vi "Servo Tracking State Machinev1.vi"(0 "Servo Positions In":cluster{"X":dbl, "Y":dbl}, 1 "Image Size":T4=enum."320x240", 5 "Target":T1, 7 "Area Limit":dbl=0.005, 9 "Found":bool) -> (4 "Servo Positions":cluster{"X":dbl, "Y":dbl}, 6 "Tracking State Info":T3)   [LabVIEW 2013]
doc: "This VI updates the servo to center the camera on the target. It uses a state based control approach to locate follow, and reacquire the target."
uses:
  <vilib>/Rock Robotics/WPI/Camera/WPI_CameraImageSize.ctl
  Control Statesv1.ctl
panel:
  in  "Upper Limit":cluster{"X":i32, "Y":i32}={"X"=169, "Y"=130}
  in  "Lower Limit":cluster{"X":i32, "Y":i32}={"X"=0, "Y"=40}
  in  "Search Speed":i32=4
  in  "Proportional (div)":cluster{"X":i32, "Y":i32}={"X"=15, "Y"=-13}
  # "Unwired tuning params for control.\nSearch speed determines how fast the\ngimbal will move when trying to acquire\na target. Too fast and you may miss the\ntarget between frames, too slow is boring.\n\nProportional(div) is the proportional constant\nexpressed as a divisor term. Adjust this higher\nif the gimbal is oscillating, lower for quicker\nresponse.\n\nThe limits are useful for keeping the gimbal in\na working range, some stick when the get near\ntheir mechanical limits. It is also useful to limit\nthe searching to avoid looking at the ceiling, etc."
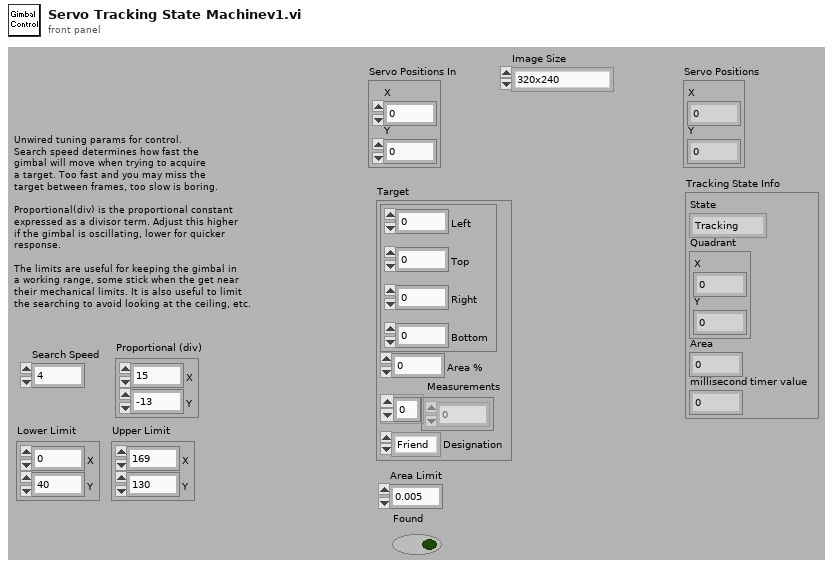
[diagram p1: front panel]
types:
  T1 = cluster{"Rectangle":cluster{"Left":i32, "Top":i32, "Right":i32, "Bottom":i32}, "Area %":dbl, "Measurements":dbl[], "Designation":enum16{"Friend", "Foe"}}
  T2 = typedef "Control Statesv1.ctl" = enum16{"Tracking", "Lost Small", "Lost-Patience", "Search-Begin", "Searching", "Lost - Edge"}
  T3 = cluster{"State":T2, "Quadrant":cluster{"X":i32, "Y":i32}, "Area":dbl, "millisecond timer value":u32}
  T4 = typedef "WPI_CameraImageSize.ctl" = enum16{"640x480", "320x240", "160x120"}
  T5 = cluster{"State":T2, "Grid Element":cluster{"X":i32, "Y":i32}, "Area":dbl, "millisecond timer value":u32}
  T6 = cluster{"Left":i32, "Top":i32, "Right":i32, "Bottom":i32}
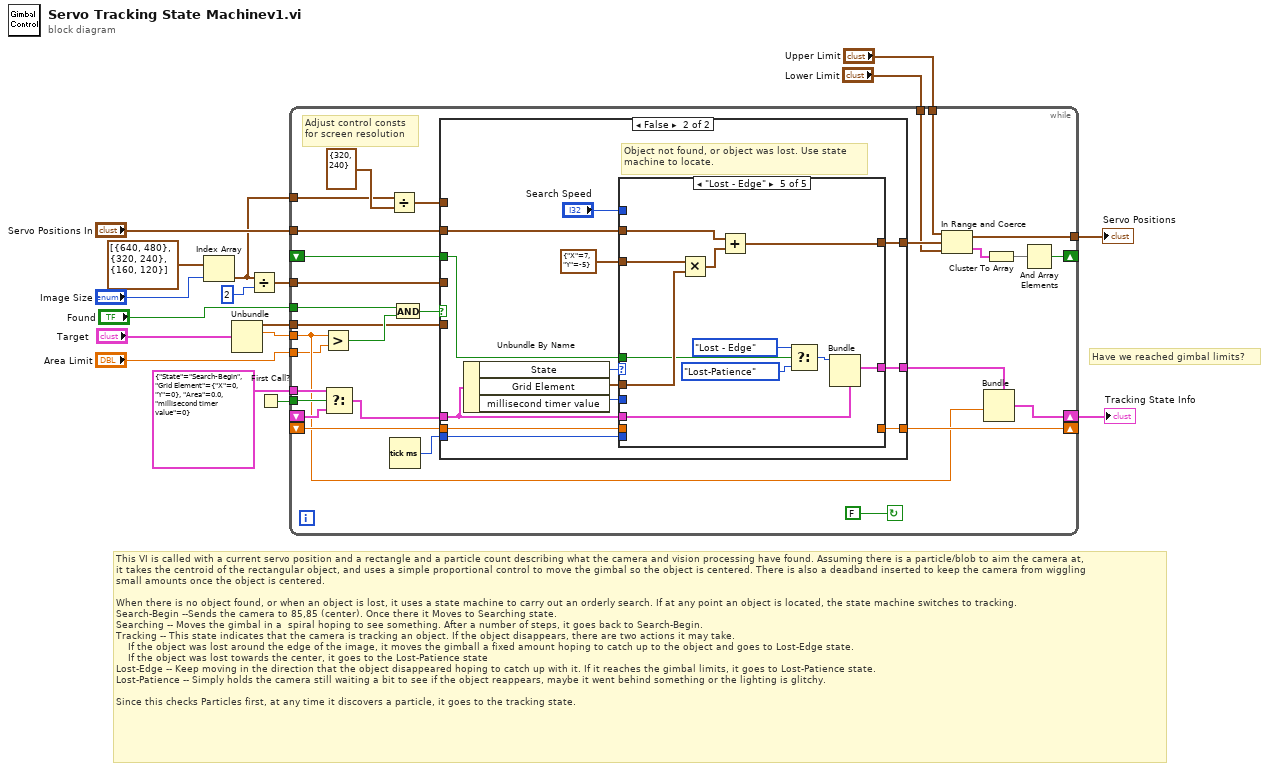
[diagram p0: block diagram]
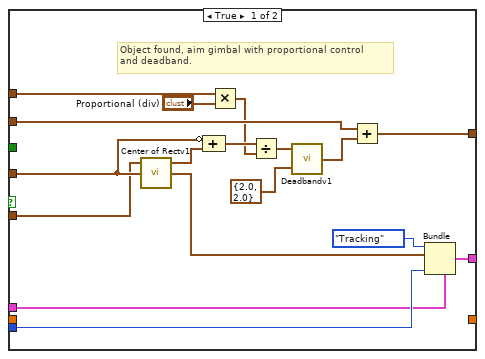
[diagram p2: hidden frame]
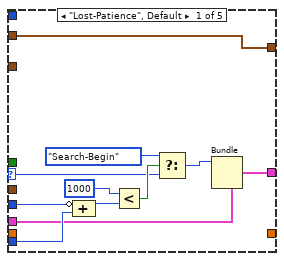
[diagram p3: hidden frame]
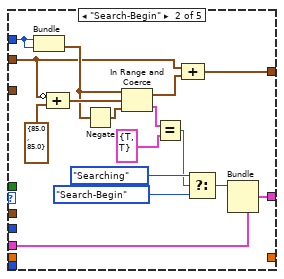
[diagram p4: hidden frame]
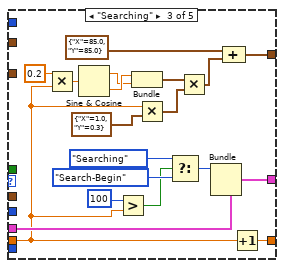
[diagram p5: hidden frame]
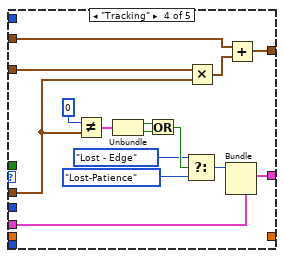
[diagram p6: hidden frame]
diagram:
  # "Have we reached gimbal limits?"
  # "This VI is called with a current servo position and a rectangle and a particle count describing what the camera and vision processing have found. Assuming there is a particle/blob to aim the camera at,\nit takes the centroid of the rectangular object, and uses a simple proportional control to move the gimbal so the object is centered. There is also a deadband inserted to keep the camera from wiggling\nsmall amounts once the object is centered.\n\nWhen there is no object found, or when an object is lost, it uses a state machine to carry out an orderly search. If at any point an object is located, the state machine switches to tracking.\nSearch-Begin --Sends the camera to 85,85 (center). Once there it Moves to Searching state.\nSearching -- Moves the gimbal in a  spiral hoping to see something. After a number of steps, it goes back to Search-Begin.\nTracking -- This state indicates that the camera is tracking an object. If the object disappears, there are two actions it may take.\n    If the object was lost around the edge of the image, it moves the gimball a fixed amount hoping to catch up to the object and goes to Lost-Edge state.\n    If the object was lost towards the center, it goes to the Lost-Patience state\nLost-Edge -- Keep moving in the direction that the object disappeared hoping to catch up with it. If it reaches the gimbal limits, it goes to Lost-Patience state.\nLost-Patience -- Simply holds the camera still waiting a bit to see if the object reappears, maybe it went behind something or the lighting is glitchy.\n\nSince this checks Particles first, at any time it discovers a particle, it goes to the tracking state."
  n1 = Index Array(array=cluster{"X":i32, "Y":i32}[] [{"X"=640, "Y"=480}, {"X"=320, "Y"=240}, {"X"=160, "Y"=120}] ("Resolutions"), index="Image Size") -> (element=w3:cluster{"X":i32, "Y":i32})
  n2 = Unbundle("Target") -> ("Rectangle"=w5:T6, "Area %"=w6:dbl)  [unwired: 2 out]
  n3 = Divide(x=w3, y=2) -> (x/y=w15:cluster{"X":dbl, "Y":dbl})
  n4 = First Call?() -> (First Call?: T/F=w10:bool)
  n5 = while {
    tunnel: w15 -> [w29]
    tunnel: [w37] -> w13
    shift-right: [w45] -> _
    shift-left: _ -> [w44]
    tunnel: "Servo Positions In" -> [w43]
    shift-right: [w26] -> w11
    shift-left: _ -> [w40]
    tunnel: w10 -> [w42]
    tunnel: T5 {"State"=enum."Search-Begin", "Grid Element"={"X"=0, "Y"=0}, "Area"=0.0, "millisecond timer value"=0} -> [w41]
    tunnel: "Lower Limit" -> [w35]
    tunnel: "Upper Limit" -> [w34]
    shift-right: [w31] -> _
    shift-left: _ -> [w30]
    tunnel: w6 -> [w24]
    tunnel: w5 -> [w23]
    tunnel: "Area Limit" -> [w22]
    tunnel: w3 -> [w19]
    tunnel: "Found" -> [w18]
    stop <- FALSE continue-if-true
    # "Adjust control consts\nfor screen resolution"
    n6 = Greater?(x=w24, y=w22) -> (0:w28:bool)
    n7 = Select(t=w41, s=w42, f=w40) -> (s? t:f=w39:T5)
    n8 = Divide(x=w19, y=cluster{"X":i32, "Y":i32} {"X"=320, "Y"=240} ("element")) -> (x/y=w21:cluster{"X":dbl, "Y":dbl})
    n9 = Tick Count (ms)() -> (millisecond timer value=w46:u32)
    n10 = And(x=w18, y=w28) -> (x .and. y?=w27:bool)
    n11 = case shown="False" w27 {
      tunnel: w29 -> [w51 _]
      tunnel: w46 -> [w59 w75]
      tunnel: [w61 w76] -> w25
      tunnel: w39 -> [w54 w68]
      tunnel: w43 -> [w60 w73]
      tunnel: [w58 w74] -> w36
      tunnel: w44 -> [_ w72]
      tunnel: [_ w71] -> w45
      tunnel: w30 -> [_ w70]
      tunnel: w23 -> [w50 _]
      tunnel: w21 -> [w47 _]
      frame True {
        # "Object found, aim gimbal with proportional control\nand deadband."
        n12 = call "Center of Rectv1.vi"("Camera Center"=w51, "Rectangle"=w50) -> ("Grid Element"=w52:cluster{"X":i32, "Y":i32}, "Center"=w53:cluster{dbl, dbl})  [unwired: 1 in, 1 out]
        n13 = Compound Arithmetic op=ADD(invert w51, w53) -> (w63:cluster{dbl, dbl})
        n14 = Multiply(x=w47, y="Proportional (div)") -> (x*y=w48:cluster{"X":dbl, "Y":dbl})
        n15 = Divide(x=w63, y=w48) -> (x/y=w56:cluster{dbl, dbl})
        n16 = call "Deadbandv1.vi"("Deadband"=cluster{dbl, dbl} {2.0, 2.0}, "Value"=w56) -> ("Value Out"=w55:cluster{dbl, dbl})
        n17 = Add(x=w60, y=w55) -> (x+y=w58:cluster{dbl, dbl})
        n18 = Bundle(cluster=w54, "State"=Control_Statesv1."Tracking", "Grid Element"=w52, "millisecond timer value"=w59) -> (w61:T5)  [unwired: 1 out]
      }
      frame False {
        # "Object not found, or object was lost. Use state\nmachine to locate."
        n19 = Unbundle By Name(w68) -> ("State"=w67:T2, "Grid Element"=w66:cluster{"X":i32, "Y":i32}, "millisecond timer value"=w65:u32)
        n20 = case shown="\"Lost - Edge\"" w67 {
          selector: w67 -> [w78 _ _ _ _]
          tunnel: [w79 w94 w109 w137 w148] -> w76
          tunnel: w68 -> [w83 w95 w110 w136 w147]
          tunnel: w65 -> [w86 _ _ _ _]
          tunnel: w75 -> [w87 _ _ _ _]
          tunnel: [w77 w96 w114 w128 w144] -> w74
          tunnel: w73 -> [w77 w97 _ w127 w145]
          tunnel: "Search Speed" -> [_ w101 _ _ _]
          tunnel: w72 -> [_ _ w105 _ _]
          tunnel: [_ _ w122 _ _] -> w71
          tunnel: w66 -> [_ _ _ w125 w143]
          tunnel: w70 -> [_ _ _ _ w139]
          tunnel: cluster{"X":i32, "Y":i32} {"X"=7, "Y"=-5} ("x") -> [_ _ _ w123 w138]
          frame "Lost-Patience", Default {
            n21 = Compound Arithmetic op=ADD(invert w86, w87) -> (w85:u32)
            n22 = Less?(x=1000, y=w85) -> (x < y?=w80:bool)
            n23 = Select(t=Control_Statesv1."Search-Begin" ("State"), s=w80, f=w78) -> (s? t:f=w82:T2)
            n24 = Bundle(cluster=w83, "State"=w82) -> (w79:T5)  [unwired: 3 out]
          }
          frame "Search-Begin" {
            n25 = Bundle("Search Speed"=w101, "Search Speed"=w101) -> (w100:cluster{"Search Speed":i32, "Search Speed":i32})  [unwired: 1 out]
            n26 = Compound Arithmetic op=ADD(invert w97, cluster{"X":dbl, "Y":dbl} {"X"=85.0, "Y"=85.0} ("Servos")) -> (w102:cluster{"X":dbl, "Y":dbl})
            n27 = Negate(x=w100) -> (-x=w99:cluster{"Search Speed":i32, "Search Speed":i32})
            n28 = In Range and Coerce(upper limit=w100, x=w102, lower limit=w99) -> (coerced(x)=w98:cluster{"X":dbl, "Y":dbl}, In Range?=w90:cluster{"X":bool, "Y":bool})
            n29 = Equal?(x=w90, y=cluster{"X":bool, "Y":bool} {"X"=TRUE, "Y"=TRUE}) -> (x = y?=w88:bool)
            n30 = Compound Arithmetic op=ADD(w97, w98) -> (w96:cluster{"X":dbl, "Y":dbl})
            n31 = Select(t=Control_Statesv1."Searching" ("State"), s=w88, f=Control_Statesv1."Search-Begin" ("State")) -> (s? t:f=w93:T2)
            n32 = Bundle(cluster=w95, "State"=w93) -> (w94:T5)  [unwired: 3 out]
          }
          frame "Searching" {
            n33 = Multiply(x=0.2, y=w105) -> (x*y=w120:dbl)
            n34 = Sine & Cosine(0:w120) -> (1:w118:dbl, 2:w119:dbl)
            n35 = Greater?(x=100, y=w105) -> (0:w107:bool)
            n36 = Bundle(w119, w118) -> (w117:cluster{dbl, dbl})  [unwired: 1 out]
            n37 = Multiply(x=w105, y=cluster{"X":dbl, "Y":dbl} {"X"=1.0, "Y"=0.3} ("Servos")) -> (x*y=w106:cluster{"X":dbl, "Y":dbl})
            n38 = Select(t=Control_Statesv1."Searching" ("State"), s=w107, f=Control_Statesv1."Search-Begin" ("State")) -> (s? t:f=w113:T2)
            n39 = Multiply(x=w117, y=w106) -> (x*y=w116:cluster{dbl, dbl})
            n40 = Bundle(cluster=w110, "State"=w113) -> (w109:T5)  [unwired: 3 out]
            n41 = Compound Arithmetic op=ADD(cluster{"X":dbl, "Y":dbl} {"X"=85.0, "Y"=85.0} ("Servos"), w116) -> (w114:cluster{dbl, dbl})
            n42 = Increment(x=w105) -> (x+1=w122:dbl)
          }
          frame "Tracking" {
            n43 = Not Equal?(x=0 ("X"), y=w125) -> (x != y?=w135:cluster{"X":bool, "Y":bool})
            n44 = Unbundle(w135) -> ("X"=w134:bool, "Y"=w133:bool)
            n45 = Or(x=w134, y=w133) -> (x .or. y?=w132:bool)
            n46 = Select(t=Control_Statesv1."Lost - Edge" ("State"), s=w132, f=Control_Statesv1."Lost-Patience" ("State")) -> (s? t:f=w129:T2)
            n47 = Multiply(x=w123, y=w125) -> (x*y=w126:cluster{"X":i32, "Y":i32})
            n48 = Bundle(cluster=w136, "State"=w129) -> (w137:T5)  [unwired: 3 out]
            n49 = Add(x=w127, y=w126) -> (x+y=w128:cluster{"X":dbl, "Y":dbl})
          }
          frame "Lost - Edge" {
            n50 = Multiply(x=w138, y=w143) -> (x*y=w146:cluster{"X":i32, "Y":i32})
            n51 = Add(x=w145, y=w146) -> (x+y=w144:cluster{"X":dbl, "Y":dbl})
            n52 = Select(t=Control_Statesv1."Lost - Edge" ("State"), s=w139, f=Control_Statesv1."Lost-Patience" ("State")) -> (s? t:f=w142:T2)
            n53 = Bundle(cluster=w147, "State"=w142) -> (w148:T5)  [unwired: 3 out]
          }
        }
      }
    }
    n54 = In Range and Coerce(upper limit=w34, x=w36, lower limit=w35) -> (coerced(x)=w37:cluster{"X":dbl, "Y":dbl}, In Range?=w33:cluster{"X":bool, "Y":bool})
    n55 = Bundle(cluster=w25, "Area"=w24) -> (w26:T5)  [unwired: 3 out]
    n56 = Cluster To Array(cluster=w33) -> (array=w32:bool[])
    n57 = And Array Elements(Boolean array=w32) -> (logical AND=w31:bool)
  }
  "Servo Positions" <- w13
  "Tracking State Info" <- w11
